vi "Example Global Variable.vi"() -> ()   [LabVIEW 2018]
uses:
  <vilib>/LabVIEW Universal Transcriptor/LabVIEW for Arduino Complex Numbers Static/ComplexNumberStatic.lvclass
  <vilib>/LabVIEW Universal Transcriptor/LabVIEW Universal Transcriptor Rotary Encoder Library/Encoder.lvclass
panel:
  out "data":refnum<class "ComplexNumberStatic.lvclass">
  out "GlobalVariableVariant":variant
  out "GlobalDoubleVariable":dbl
  in  "GlobalVarArrayString 2":string[](array[string])
  out "GlobalVarArrayString":string[](array[string])
  out "error out":errorcluster
  in  "error in (no error)":errorcluster
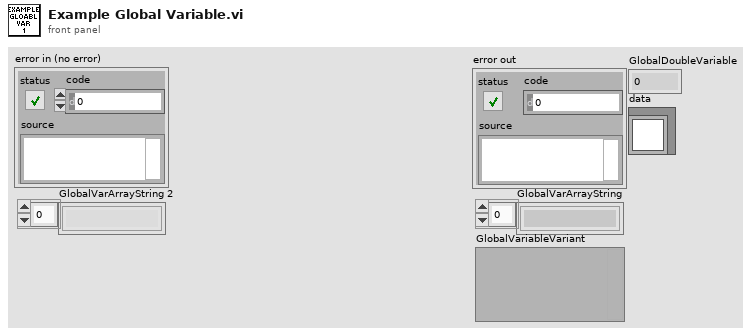
[diagram p1: front panel]
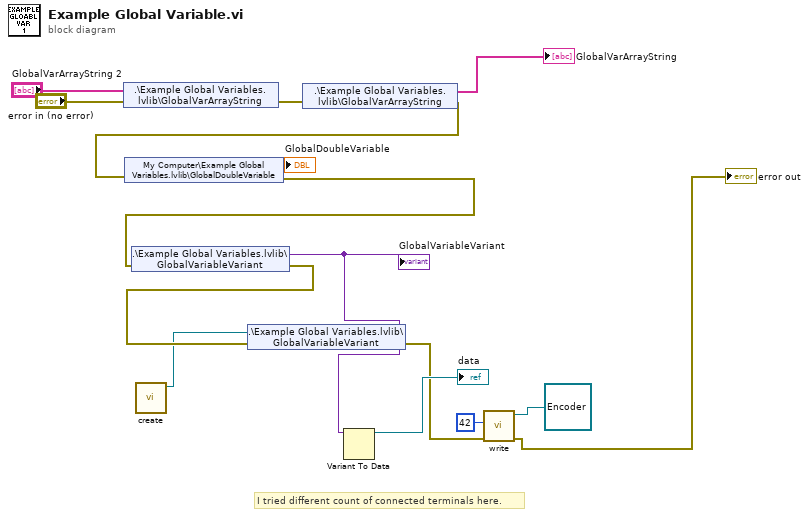
[diagram p0: block diagram]
diagram:
  # "I tried different count of connected terminals here."
  n1 = shared-variable ".\\Example Global Variables.lvlib\\GlobalVarArrayString"("GlobalVarArrayString 2", error in="error in (no error)") -> (error out=w13:errorcluster)
  n2 = call <vilib>:"create.vi"() -> ("Encoder in"=w7:refnum<class "Encoder.lvclass">)  [unwired: 10 in, 1 out]
  n3 = shared-variable ".\\Example Global Variables.lvlib\\GlobalVarArrayString"(error in=w13) -> (→"GlobalVarArrayString":string[], error out=w11:errorcluster)
  n4 = shared-variable "My Computer\\Example Global Variables.lvlib\\GlobalDoubleVariable"(error in=w11) -> (→"GlobalDoubleVariable":dbl, error out=w9:errorcluster)
  n5 = shared-variable ".\\Example Global Variables.lvlib\\GlobalVariableVariant"(error in=w9) -> (w6:variant, error out=w8:errorcluster)
  "GlobalVariableVariant" <- w6
  n6 = shared-variable ".\\Example Global Variables.lvlib\\GlobalVariableVariant"(w7, error in=w8) -> (error out=w1:errorcluster)
  n7 = Variant To Data(Variant=w6) -> (data=→"data":refnum<class "ComplexNumberStatic.lvclass">)  [unwired: 2 in, 1 out]
  n8 = call <vilib>:"write.vi"("error in (no error)"=w1, "value"=42, "Encoder in"=refnum<class "Encoder.lvclass"> refnum) -> ("error out"=→"error out":errorcluster)  [unwired: 7 in]
